vi "encoderdirection1.vi"() -> ()   [LabVIEW 2016]
panel:
  out "String":string
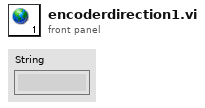
[diagram p1: front panel]
diagram:
